vi "Generate New Log Path Event.vi"(10 "error in (no error)":errorcluster, 11 "New Log Path":path) -> (2 "error out":errorcluster)   [LabVIEW 2020]
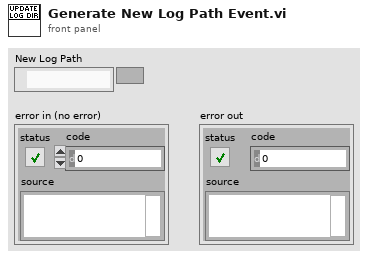
[diagram p1: front panel]
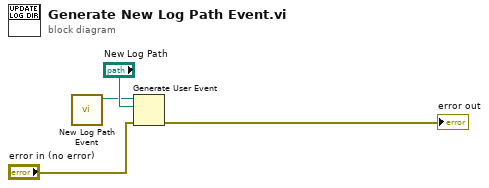
[diagram p0: block diagram]
diagram:
  n1 = call "New Log Path Event.vi"() -> ("New Log Path"=w1:refnum<user-event>)  [unwired: 11 in]
  n2 = Generate User Event(user event=w1, event data cluster="New Log Path", error in="error in (no error)") -> (error out=→"error out":errorcluster)  [unwired: 1 in, 1 out]
